vi "Controller LNLS Control FOFB Configuration Communication Loop.vi"(7 "Sync Objects":T3, 8 "error in (no error)":errorcluster, 11 "FOFB Configuration":T6={"FOFB Parameters"={"Network"={"FOFB Controller IP"="", "LNLS Control Network IP"="", "LNLS Control Network Power Supplies TCP Port"=0, "LNLS Control Network FOFB Configuration TCP Port"=0, "LNLS Control Network BPMs TCP Port"=0, "Monitoring Data TCP Port"=0, "Fast Archiver TCP Port"=0, "Fast Command TCP Port"=0, "TCP Listening Timeout"=0}, "Fast Acquisition"={"Sampling Period"=0, "Data Buffer Size"=0, "Monitoring Period"=0}, "Acquisition Network"=[], "Actuation Network"=[]}, "Number of Acquisition Chassis"=0, "Number of Actuation Chassis"=0, "Number of BPM Readings"=0, "BPM Reading Names"=[], "Selected BPM Readings"=[0, 1, 2, 3, 4, 5, 6, 7, 8, 9, 10, 11, 12, 13, 14, 15, 16, 17, 18, 19, 20, 21, 22, 23, 24, 25, 26, 27, 28, 29, 30, 31, 32, 33, 34, 35, 36, 37, 38, 39, 40, 41, 42, 43, 44, 45, 46, 47, 48, 49], "Number of Correctors"=0, "Corrector Names"=[], "Selected Correctors"=[0, 1, 2, 3, 4, 5, 6, 7, 8, 9, 10, 11, 12, 13, 14, 15, 16, 17, 18, 19, 20, 21, 22, 23, 24, 25, 26, 27, 28, 29, 30, 31, 32, 33, 34, 35, 36, 37, 38, 39, 40, 41, 42, 43, 44, 45, 46, 47, 48, 49], "Response Matrix"=[], "Reference Orbit"=[], "Correction Matrix"=[], "FPGA Filter Sets"=[], "Acquisition Chassis Names"=[], "Actuation Chassis Names"=[], "Acquisition Variables"=[], "Actuation Variables"=[], "PS Matrix Mapping"=[], "Inverse PS Matrix Mapping"=[], "BPM Matrix Mapping"=[], "Inverse BPM Matrix Mapping"=[], "BPM Planes"=[], "Corrector Planes"=[]}) -> (0 "error out":errorcluster)   [LabVIEW 2011, in "Controller VIs.lvlib"]
uses:
  Controller VIs.lvlib
  Types Definitions/Type FOFB Configuration.ctl
  Types Definitions/Type FOFB Parameters.ctl
  Types Definitions/Type Network Configuration.ctl
  Types Definitions/Type FA Configuration.ctl
  Types Definitions/Type Acquisition Network Configuration.ctl
  Types Definitions/Type Actuation Network Configuration.ctl
  Types Definitions/Type Synchronization Objects.ctl
  Types Definitions/Type Blocking Synchronization Objects.ctl
  Types Definitions/Type Monitoring Data.ctl
  Types Definitions/Type Operation Mode State.ctl
  Types Definitions/Type Diagnostics Data.ctl
  Types Definitions/Type CPU Loads Array.ctl
  Types Definitions/Type CPU Loads.ctl
  Types Definitions/Type Non-blocking Synchronization Objects.ctl
  Types Definitions/Type FOFB Variables.ctl
  Types Definitions/Type Actuation State.ctl
  Types Definitions/Type Control FOFB Configuration In.ctl
  Types Definitions/Type TCP State.ctl
  <vilib>/Platform/TimedLoop/XDataNode/timing_clust.ctl
  <vilib>/Platform/TimedLoop/XDataNode/nitl_modes.ctl
  <vilib>/Platform/TimedLoop/XDataNode/wakeup.ctl
  Controller Global Variables/LNLS Control FOFB Configuration In.vi
  Controller Global Variables/LNLS Control FOFB Configuration Out.vi
  <vilib>/Platform/TimedLoop/XDataNode/XDataNode.xnode
  LNLS Control VIs.lvlib
  Misc VIs.lvlib
  Controller Global Variables.lvlib
  <vilib>/Platform/TimedLoop/XDataNode/XDNodeRunTimeDep.lvlib
  Type Definitions.lvlib
  <vilib>/real-time/NI_Real-Time Libraries.lvlib
  <vilib>/real-time/rtutility.llb/RT Restart Target (Self).vi
panel:
  in  "FOFB Configuration":T1={"Status"=0, "Operation Mode"=enum."Manual Mode", "Horizontal Gain"=0.0, "Vertical Gain"=0.0, "Selected Reference Orbit"=0, "Selected Correction Matrix"=0, "Selected FPGA Filters"=0, "Horizontal Distortion Threshold"=0.0, "Vertical Distortion Threshold"=0.0, "Fast Command Enabled"=FALSE, "Update Reference Orbit"=FALSE, "Update Contoller Configuration"=FALSE}
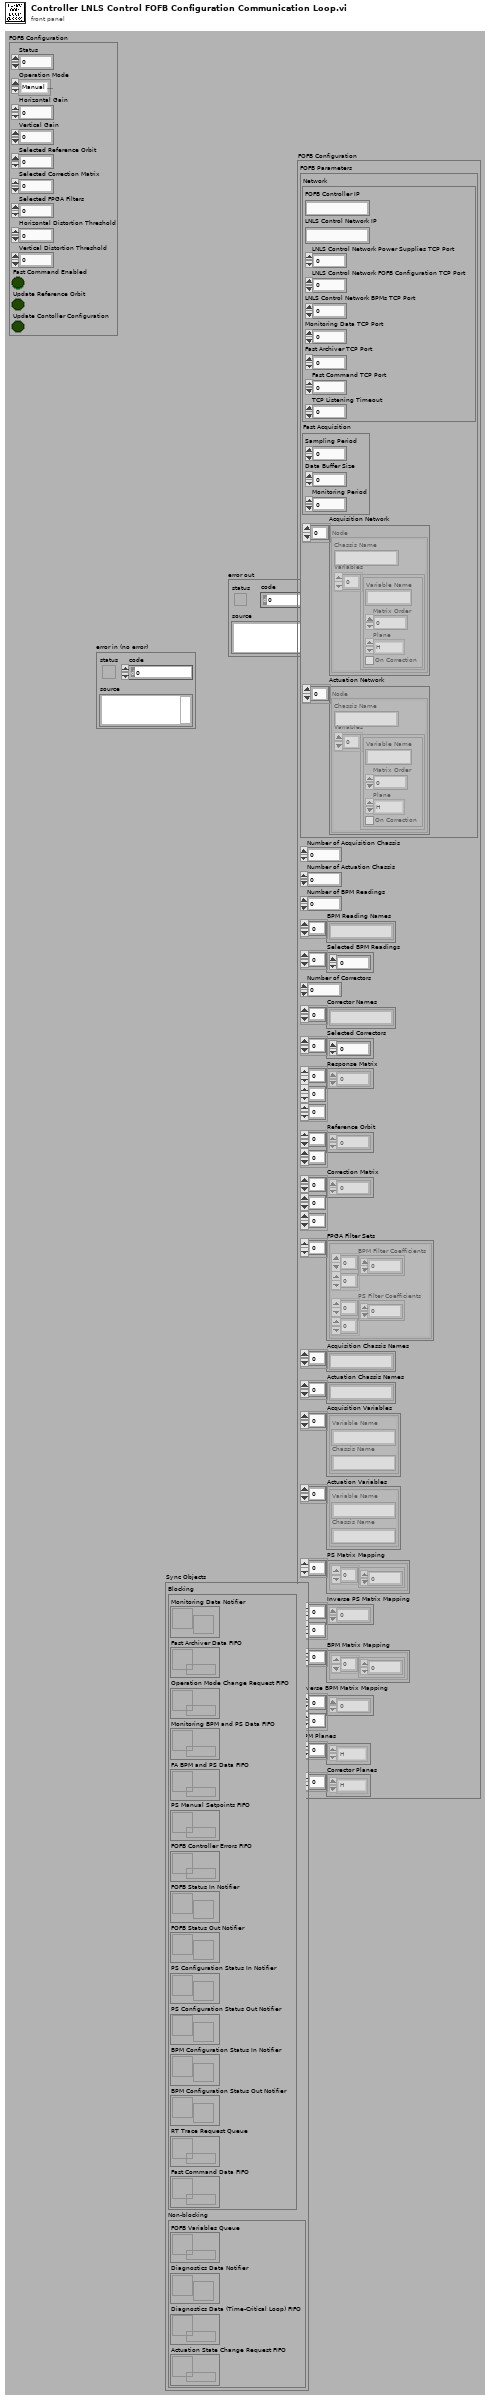
[diagram p1: front panel]
types:
  T1 = typedef "Type Definitions.lvlib/Type Control FOFB Configuration In.ctl" = cluster{"Status":u16, "Operation Mode":T2, "Horizontal Gain":sgl, "Vertical Gain":sgl, "Selected Reference Orbit":i32, "Selected Correction Matrix":i32, "Selected FPGA Filters":i32, "Horizontal Distortion Threshold":sgl, "Vertical Distortion Threshold":sgl, "Fast Command Enabled":bool, "Update Reference Orbit":bool, "Update Contoller Configuration":bool}
  T2 = typedef "Type Definitions.lvlib/Type Operation Mode State.ctl" = enum8{"Idle Mode", "Manual Mode", "FOFB Mode"}
  T3 = typedef "Type Definitions.lvlib/Type Synchronization Objects.ctl" = cluster{"Blocking":T4, "Non-blocking":T5}
  T4 = typedef "Type Definitions.lvlib/Type Blocking Synchronization Objects.ctl" = cluster{"Monitoring Data Notifier":refnum<notifier>, "Fast Archiver Data FIFO":refnum<queue>, "Operation Mode Change Request FIFO":refnum<k33>, "Monitoring BPM and PS Data FIFO":refnum<k33>, "FA BPM and PS Data FIFO":refnum<k33>, "PS Manual Setpoints FIFO":refnum<k33>, "FOFB Controller Errors FIFO ":refnum<k33>, "FOFB Status In Notifier":refnum<notifier>, "FOFB Status Out Notifier":refnum<notifier>, "PS Configuration Status In Notifier":refnum<notifier>, "PS Configuration Status Out Notifier":refnum<notifier>, "BPM Configuration Status In Notifier":refnum<notifier>, "BPM Configuration Status Out Notifier":refnum<notifier>, "RT Trace Request Queue":refnum<queue>, "Fast Command Data FIFO":refnum<k33>}
  T5 = typedef "Type Definitions.lvlib/Type Non-blocking Synchronization Objects.ctl" = cluster{"FOFB Variables Queue":refnum<queue>, "Diagnostics Data Notifier":refnum<notifier>, "Diagnostics Data (Time-Critical Loop) FIFO":refnum<k33>, "Actuation State Change Request FIFO":refnum<k33>}
  T6 = typedef "Type Definitions.lvlib/Type FOFB Configuration.ctl" = cluster{"FOFB Parameters":T7, "Number of Acquisition Chassis":i32, "Number of Actuation Chassis":i32, "Number of BPM Readings":i32, "BPM Reading Names":string[], "Selected BPM Readings":u32[], "Number of Correctors":i32, "Corrector Names":string[], "Selected Correctors":u32[], "Response Matrix":dbl[][][], "Reference Orbit":dbl[][], "Correction Matrix":dbl[][][], "FPGA Filter Sets":cluster{"BPM Filter Coefficients":dbl[][], "PS Filter Coefficients":dbl[][]}[], "Acquisition Chassis Names":string[], "Actuation Chassis Names":string[], "Acquisition Variables":cluster{"Variable Name":string, "Chassis Name":string}[], "Actuation Variables":cluster{"Variable Name":string, "Chassis Name":string}[], "PS Matrix Mapping":cluster{u32[]}[], "Inverse PS Matrix Mapping":u32[][], "BPM Matrix Mapping":cluster{u32[]}[], "Inverse BPM Matrix Mapping":u32[][], "BPM Planes":enum8{"H", "V"}[], "Corrector Planes":enum8{"H", "V"}[]}
  T7 = typedef "Type Definitions.lvlib/Type FOFB Parameters.ctl" = cluster{"Network":T8, "Fast Acquisition":T9, "Acquisition Network":T10, "Actuation Network":T11}
  T8 = typedef "Type Definitions.lvlib/Type Network Configuration.ctl" = cluster{"FOFB Controller IP":string, "LNLS Control Network IP":string, "LNLS Control Network Power Supplies TCP Port":u16, "LNLS Control Network FOFB Configuration TCP Port":u16, "LNLS Control Network BPMs TCP Port":u16, "Monitoring Data TCP Port":u16, "Fast Archiver TCP Port":u16, "Fast Command TCP Port":u16, "TCP Listening Timeout":i32}
  T9 = typedef "Type Definitions.lvlib/Type FA Configuration.ctl" = cluster{"Sampling Period":u32, "Data Buffer Size":u32, "Monitoring Period":u32}
  T10 = typedef "Type Definitions.lvlib/Type Acquisition Network Configuration.ctl" = cluster{"Chassis Name":string, "Variables":cluster{"Variable Name":string, "Matrix Order":u32, "Plane":enum8{"H", "V"}, "On Correction":bool}[]}[]
  T11 = typedef "Type Definitions.lvlib/Type Actuation Network Configuration.ctl" = cluster{"Chassis Name":string, "Variables":cluster{"Variable Name":string, "Matrix Order":u32, "Plane":enum8{"H", "V"}, "On Correction":bool}[]}[]
  T12 = typedef "Type Definitions.lvlib/Type TCP State.ctl" = enum16{"Idle", "Wait Connection", "Read Data", "Process Data", "Write Data", "Close Connection"}
  T13 = typedef "XDNodeRunTimeDep.lvlib/timing_clust.ctl" = cluster{"Expected End [f-1]":u64, "Actual End [f-1]":u64, "Finished Late? [f-1]":bool, "Expected End [i-1]":u64, "Actual End [i-1]":u64, "Finished Late? [i-1]":bool, "Expected Start [i]":u64, "Actual Start [i]":u64, "Expected Start [f]":u64, "Actual Start [f]":u64, "Source Name":string, "Structure Name":string, "Period":i64, "Deadline":i64, "Offset":i64, "Start":i64, "Priority":i32, "Timeout":i32, "Mode":T14, "Wakeup Reason":T15, "Error":errorcluster, "Source Type":string, "Secondary Source Type":string, "Global End Time":u64, "Global Start Time":u64, "Frame Duration":u64, "Iteration Duration":u64, "Assigned CPU":i32, "I/O Scan Engine Mode":u32}
  T14 = typedef "XDNodeRunTimeDep.lvlib/nitl_modes.ctl" = enum32{"No Change", "Process missed periods, maintain original phase", "Discard missed periods, maintain original phase", "Process missed periods, ignore original phase", "Discard missed periods, ignore original phase"}
  T15 = typedef "XDNodeRunTimeDep.lvlib/wakeup.ctl" = enum32{"Normal", "Aborted", "Asynchronous wakeup", "Timing source error", "Timed loop error", "Timeout"}
  T16 = typedef "Type Definitions.lvlib/Type Control FOFB Configuration Out.ctl" = cluster{"Status":u16, "Operation Mode":T2, "Horizontal Gain":sgl, "Vertical Gain":sgl, "Selected Reference Orbit":i32, "Selected Correction Matrix":i32, "Selected FPGA Filters":i32, "Horizontal Distortion Threshold":sgl, "Vertical Distortion Threshold":sgl, "Timestamp":dbl}
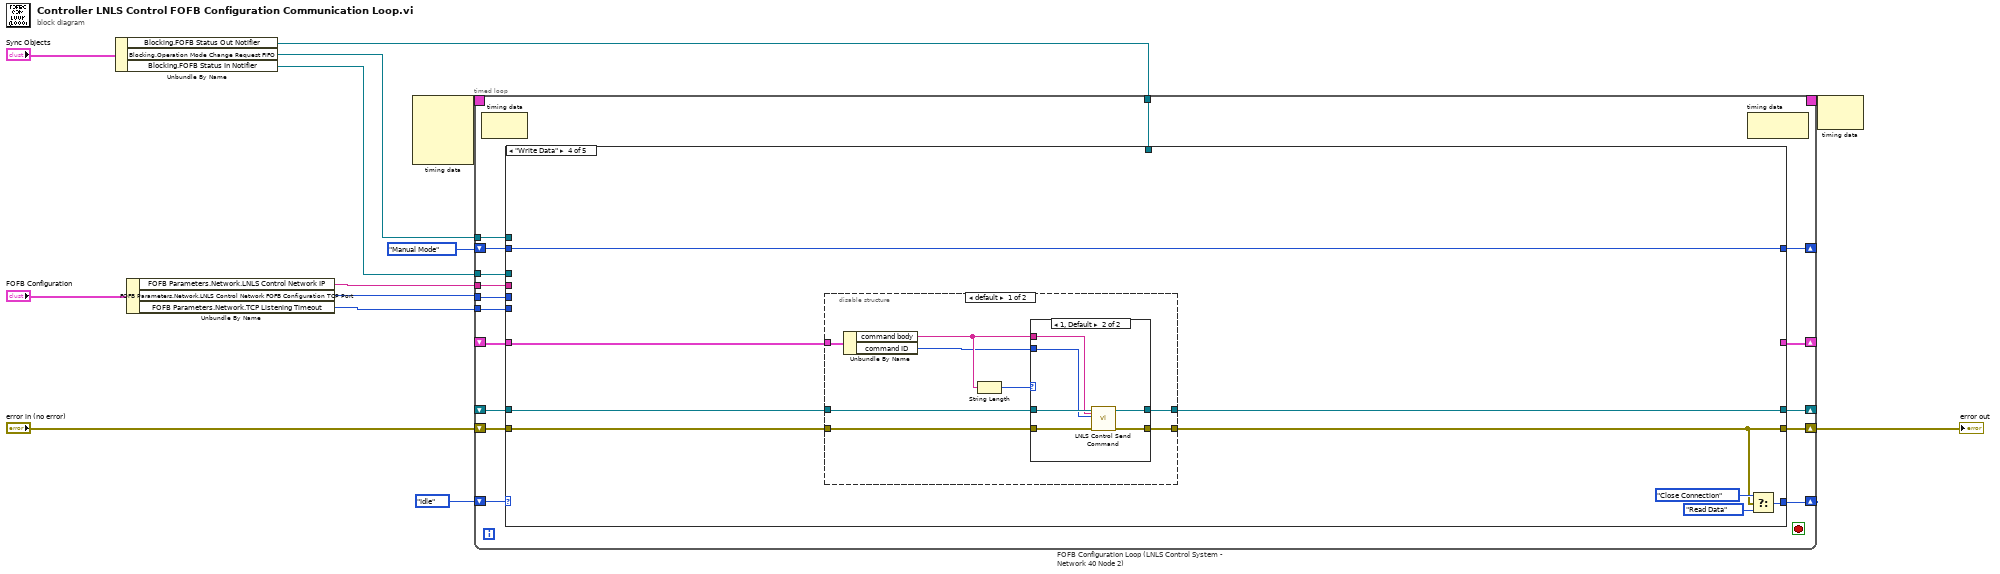
[diagram p0: block diagram]
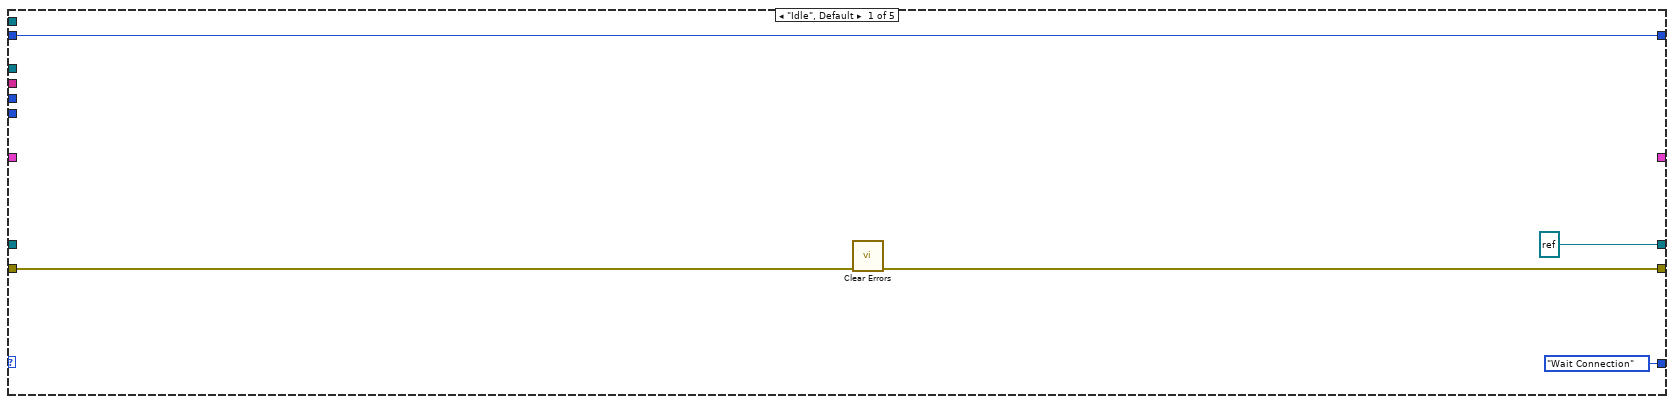
[diagram p2: hidden frame]
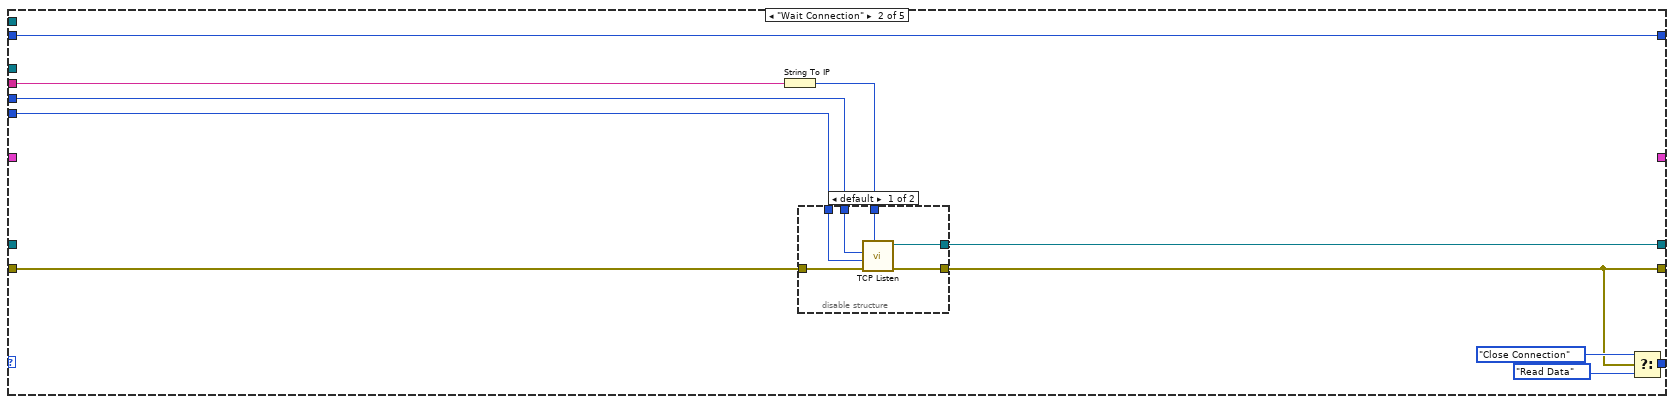
[diagram p3: hidden frame]
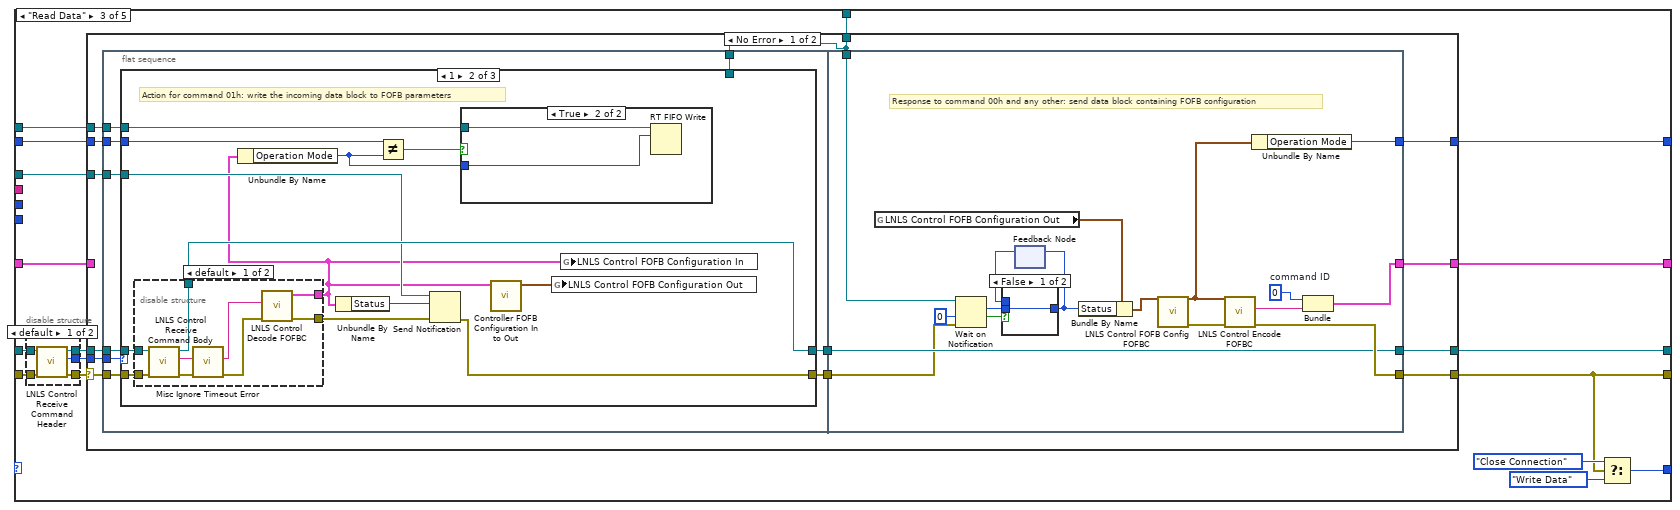
[diagram p5: hidden frame]
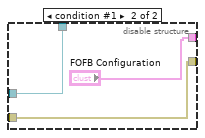
[diagram p8: hidden frame]
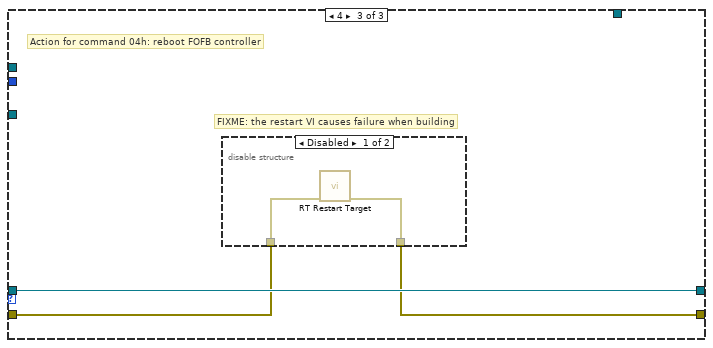
[diagram p9: hidden frame]
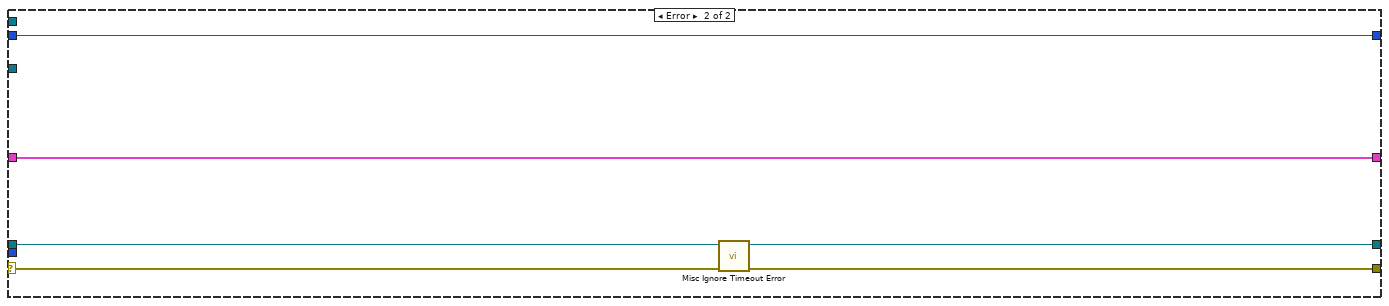
[diagram p12: hidden frame]
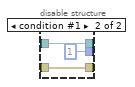
[diagram p13: hidden frame]
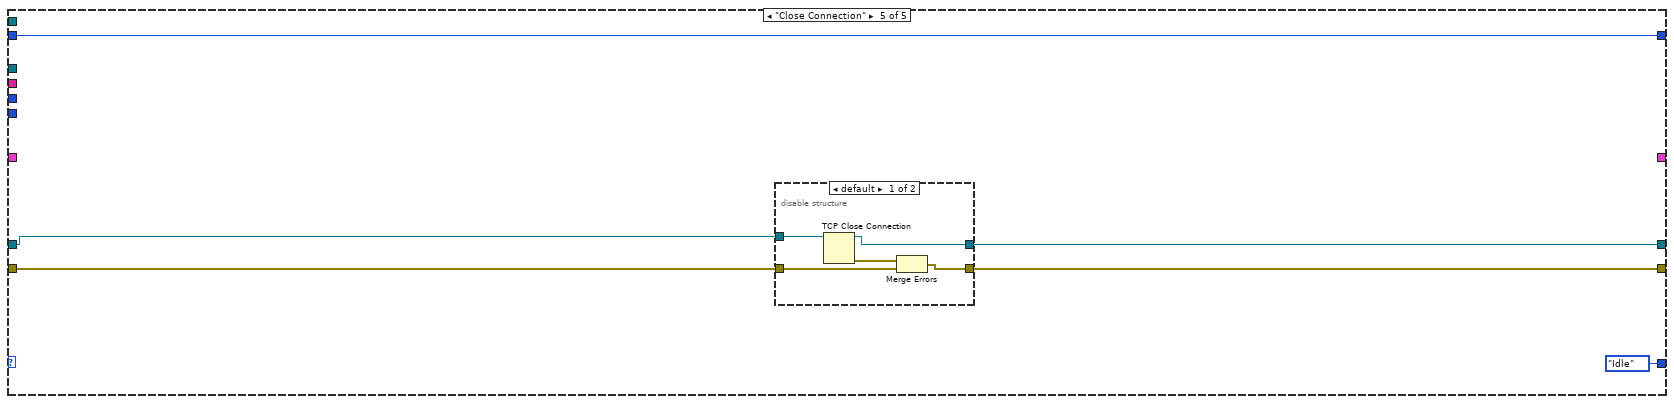
[diagram p16: hidden frame]
diagram:
  n1 = Unbundle By Name("Sync Objects") -> ("Blocking.FOFB Status Out Notifier"=w1:refnum<notifier>, "Blocking.Operation Mode Change Request FIFO"=w6:refnum<k33>, "Blocking.FOFB Status In Notifier"=w2:refnum<notifier>)
  n2 = Unbundle By Name("FOFB Configuration") -> ("FOFB Parameters.Network.LNLS Control Network IP"=w9:string, "FOFB Parameters.Network.LNLS Control Network FOFB Configuration TCP Port"=w8:u16, "FOFB Parameters.Network.TCP Listening Timeout"=w7:i32)
  n3 = node-c288() -> (w5:T13)  [unwired: 4 in]
  n4 = timed-loop "FOFB Configuration Loop (LNLS Control System - Network 40 Node 2)" {
    shift-right: [w28] -> _
    shift-left: Type_TCP_State."Idle" ("f") -> [w30]
    shift-right: [w29] -> _
    shift-left: _ -> [w27]
    shift-right: [w15] -> w12
    shift-left: "error in (no error)" -> [w24]
    shift-right: [w26] -> _
    shift-left: _ -> [w25]
    tunnel: w9 -> [w23]
    tunnel: w8 -> [w22]
    tunnel: w7 -> [w21]
    tunnel: w6 -> [w20]
    shift-right: [w18] -> _
    shift-left: Type_Operation_Mode_State."Manual Mode" ("Operation Mode") -> [w19]
    timing: w5 -> [_]
    timing-out: [_] -> w4
    tunnel: w1 -> [w17]
    tunnel: w2 -> [w16]
    stop <- _ stop-if-true
    n5 = node-c288() -> ()  [unwired: 1 in, 1 out]
    n6 = case shown="\"Write Data\"" w30 {
      tunnel: [refnum<k5> refnum ("connection ID") w43 w70 w160 w189] -> w29
      tunnel: [w31 w37 w60 w162 w185] -> w15
      tunnel: [Type_TCP_State."Wait Connection" w46 w69 w164 Type_TCP_State."Idle"] -> w28
      tunnel: w27 -> [_ _ w67 w161 w190]
      tunnel: w24 -> [w32 w38 w68 w163 w186]
      tunnel: [_ _ w64 _ _] -> w26
      tunnel: w25 -> [_ _ w62 w159 _]
      tunnel: w23 -> [_ w41 _ _ _]
      tunnel: w22 -> [_ w40 _ _ _]
      tunnel: w21 -> [_ w36 _ _ _]
      tunnel: w20 -> [_ _ w58 _ _]
      tunnel: w19 -> [w33 w39 w57 w158 w187]
      tunnel: [w33 w39 w56 w158 w187] -> w18
      tunnel: w17 -> [_ _ w55 _ _]
      tunnel: w16 -> [_ _ w54 _ _]
      frame "Idle", Default {
        n7 = call <vilib>:"Clear Errors.vi"("error in (no error)"=w32) -> ("error out"=w31:errorcluster)  [unwired: 6 in]
      }
      frame "Wait Connection" {
        n8 = String To IP(1:w41) -> (0:w42:u32)
        n9 = disable-structure shown="default" {
          disable-tunnel: [w52 _] -> w43
          disable-tunnel: w42 -> [w51 _]
          disable-tunnel: w40 -> [w50 _]
          disable-tunnel: w38 -> [w49 w53]
          disable-tunnel: [w48 w53] -> w37
          disable-tunnel: w36 -> [w47 _]
          frame condition #0 (active) {
            n10 = call <vilib>:"TCP Listen.vi"("net address"=w51, "error in (no error)"=w49, "timeout ms (wait forever: -1)"=w47, "port"=w50) -> ("error out"=w48:errorcluster, "connection ID"=w52:refnum<k5>)  [unwired: 3 in, 3 out]
          }
          frame condition #1 {
          }
        }
        n11 = Select(t=Type_TCP_State."Close Connection", s=w37, f=Type_TCP_State."Read Data") -> (s? t:f=w46:T12)
      }
      frame "Read Data" {
        n12 = disable-structure shown="default" {
          disable-tunnel: w68 -> [w154 w155]
          disable-tunnel: w67 -> [w153 w156]
          disable-tunnel: [w152 w156] -> w66
          disable-tunnel: [w151 w155] -> w63
          disable-tunnel: [w150 u8 1 ("command ID")] -> w59
          frame condition #0 (active) {
            n13 = call "LNLS Control Receive Command Header.vi"("error in (no error)"=w154, "connection ID"=w153) -> ("error out"=w151:errorcluster, "command ID"=w150:u8, "connection ID out"=w152:refnum<k5>)  [unwired: 7 in]
          }
          frame condition #1 {
          }
        }
        n14 = case shown="No Error" w63 {
          selector: w63 -> [w78 w147]
          tunnel: [w83 w149] -> w70
          tunnel: [w82 w146] -> w60
          tunnel: w66 -> [w81 w149]
          tunnel: w59 -> [w80 _]
          tunnel: [w79 w148] -> w64
          tunnel: w62 -> [_ w148]
          tunnel: w58 -> [w77 _]
          tunnel: w57 -> [w76 w145]
          tunnel: [w75 w145] -> w56
          tunnel: w55 -> [w71 _]
          tunnel: w54 -> [w74 _]
          frame No Error {
            n15 = flat-sequence {
              tunnel: [w92] -> w73
              tunnel: [w91] -> w72
              tunnel: w81 -> [w90]
              tunnel: w80 -> [w89]
              tunnel: w78 -> [w88]
              tunnel: w77 -> [w87]
              tunnel: w76 -> [w86]
              tunnel: w74 -> [w85]
              tunnel: w71 -> [w84]
              tunnel: [w141] -> w83
              tunnel: w73 -> [w141]
              tunnel: [w142] -> w82
              tunnel: w72 -> [w133]
              tunnel: [w140] -> w79
              tunnel: [w137] -> w75
              tunnel: w71 -> [w134]
              frame #0 {
                n16 = case shown="1" w89 {
                  tunnel: w88 -> [w94 w106 w122]
                  tunnel: [w94 w101 w121] -> w91
                  tunnel: [w93 w105 w123] -> w92
                  tunnel: w90 -> [w93 w107 w123]
                  tunnel: w87 -> [_ w104 _]
                  tunnel: w86 -> [_ w103 _]
                  tunnel: w85 -> [_ w102 _]
                  tunnel: w84 -> [_ _ _]
                  frame 0, Default {
                  }
                  frame 1 {
                    # "Action for command 01h: write the incoming data block to FOFB parameters"
                    n17 = disable-structure shown="default" {
                      disable-tunnel: w107 -> [w117 w119]
                      disable-tunnel: w106 -> [w116 w120]
                      disable-tunnel: [w115 w119] -> w105
                      disable-tunnel: [w111 w120] -> w99
                      disable-tunnel: [w110 "FOFB Configuration"] -> w97
                      frame condition #0 (active) {
                        n18 = call "LNLS Control Receive Command Body.vi"("error in (no error)"=w116, "connection ID"=w117) -> ("error out"=w114:errorcluster, "command body"=w112:string, "connection ID out"=w115:refnum<k5>)  [unwired: 6 in, 1 out]
                        n19 = call "Misc Ignore Timeout Error.vi"("error in (no error)"=w114) -> ("error out"=w113:errorcluster)  [unwired: 9 in, 1 out]
                        n20 = call "LNLS Control Decode FOFBC.vi"("error in (no error)"=w113, "command body"=w112) -> ("error out"=w111:errorcluster, "LNLS Control FOFB Configuration In"=w110:T1)  [unwired: 8 in]
                      }
                      frame condition #1 {
                      }
                    }
                    n21 = Unbundle By Name(w97) -> ("Operation Mode"=w95:T2)
                    n22 = Unbundle By Name(w97) -> ("Status"=w100:u16)
                    n23 = Not Equal?(x=w103, y=w95) -> (x != y?=w96:bool)
                    n24 = Send Notification(notification=w100, notifier=w102, error in (no error)=w99) -> (error out=w101:errorcluster)  [unwired: 1 out]
                    n25 = case shown="True" w96 {
                      tunnel: w104 -> [_ w109]
                      tunnel: w95 -> [_ w108]
                      frame False {
                      }
                      frame True {
                        n26 = RT FIFO Write(0:w109, 1:w108) -> ()  [unwired: 3 in, 4 out]
                      }
                    }
                    n27 = call "Controller FOFB Configuration In to Out.vi"("LNLS Control FOFB Configuration In"=w97) -> ("LNLS Control FOFB Configuration Out"=w98:T16)  [unwired: 10 in]
                    n28 = global write "LNLS Control FOFB Configuration Out.vi" "LNLS Control FOFB Configuration Out"(w98) -> ()
                    n29 = global write "LNLS Control FOFB Configuration In.vi" "LNLS Control FOFB Configuration In"(w97) -> ()
                  }
                  frame 4 {
                    # "FIXME: the restart VI causes failure when building"
                    # "Action for command 04h: reboot FOFB controller"
                    n30 = disable-structure shown="Disabled" {
                      disable-tunnel: w122 -> [w125 _]
                      disable-tunnel: [w124 _] -> w121
                      frame Disabled {
                        n31 = call-poly <vilib>:"RT Restart Target.vi"("error in (no error)"=w125) -> ("error out"=w124:errorcluster)  [unwired: 10 in]
                      }
                      frame Enabled {
                      }
                    }
                  }
                }
              }
              frame #1 {
                w138 = u8 0  # command ID
                # "Response to command 00h and any other: send data block containing FOFB configuration"
                n32 = global read "LNLS Control FOFB Configuration Out.vi" "LNLS Control FOFB Configuration Out"() -> (w130:T16)
                n33 = Wait on Notification(notifier=w134, timeout in ms (-1)=0, error in (no error)=w133) -> (notification=w128:u16, timed out?=w129:bool)  [unwired: 1 in, 2 out]
                n34 = feedback #1() -> (w127:u16)  [unwired: 1 in]
                n35 = case shown="False" w129 {
                  tunnel: [w143 w144] -> w126
                  tunnel: w128 -> [w143 _]
                  tunnel: w127 -> [_ w144]
                  frame False {
                  }
                  frame True {
                  }
                }
                n36 = feedback-in #1(w126) -> ()
                n37 = Bundle By Name(cluster=w130, "Status"=w126) -> (w132:T16)
                n38 = call "LNLS Control FOFB Config FOFBC.vi"("LNLS Control FOFB Configuration Out"=w132) -> ("error out"=w136:errorcluster, "PFOFBC Data"=w135:T16)  [unwired: 9 in]
                n39 = call "LNLS Control Encode FOFBC.vi"("error in (no error)"=w136, "PFOFBC Data"=w135) -> ("error out"=w142:errorcluster, "command body"=w139:string)  [unwired: 8 in]
                n40 = Unbundle By Name(w135) -> ("Operation Mode"=w137:T2)
                n41 = Bundle("command ID"=w138, "command body"=w139) -> (w140:cluster{"command ID":u8, "command body":string})  [unwired: 1 in]
              }
            }
          }
          frame Error {
            n42 = call "Misc Ignore Timeout Error.vi"("error in (no error)"=w147) -> ("error out"=w146:errorcluster)  [unwired: 9 in, 1 out]
          }
        }
        n43 = Select(t=Type_TCP_State."Close Connection", s=w60, f=Type_TCP_State."Write Data") -> (s? t:f=w69:T12)
      }
      frame "Write Data" {
        n44 = disable-structure shown="default" {
          disable-tunnel: w163 -> [w171 w184]
          disable-tunnel: [w170 w184] -> w162
          disable-tunnel: w161 -> [w169 w183]
          disable-tunnel: [w168 w183] -> w160
          disable-tunnel: w159 -> [w167 _]
          frame condition #0 (active) {
            n45 = Unbundle By Name(w167) -> ("command body"=w174:string, "command ID"=w172:u8)
            n46 = String Length(string=w174) -> (length=w173:i32)
            n47 = case shown="1, Default" w173 {
              tunnel: w169 -> [w175 w182]
              tunnel: w171 -> [w176 w181]
              tunnel: [w176 w180] -> w170
              tunnel: [w175 w179] -> w168
              tunnel: w174 -> [_ w178]
              tunnel: w172 -> [_ w177]
              frame 0 {
              }
              frame 1, Default {
                n48 = call "LNLS Control Send Command.vi"("command body"=w178, "error in (no error)"=w181, "command ID"=w177, "connection ID"=w182) -> ("error out"=w180:errorcluster, "connection ID out"=w179:refnum<k5>)  [unwired: 6 in]
              }
            }
          }
          frame condition #1 {
          }
        }
        n49 = Select(t=Type_TCP_State."Close Connection", s=w162, f=Type_TCP_State."Read Data") -> (s? t:f=w164:T12)
      }
      frame "Close Connection" {
        n50 = disable-structure shown="default" {
          disable-tunnel: w190 -> [w195 w196]
          disable-tunnel: [w194 w196] -> w189
          disable-tunnel: w186 -> [w192 w197]
          disable-tunnel: [w191 w197] -> w185
          frame condition #0 (active) {
            n51 = TCP Close Connection(connection ID=w195) -> (connection ID out=w194:refnum<k5>, error out=w193:errorcluster)  [unwired: 2 in]
            n52 = Merge Errors(w193, w192) -> (w191:errorcluster)
          }
          frame condition #1 {
          }
        }
      }
    }
    n53 = node-c288() -> ()  [unwired: 1 in, 1 out]
  }
  "error out" <- w12
  n54 = node-c288(w4) -> ()  [unwired: 1 out]
